vi "lab10.vi"() -> ()   [LabVIEW 2018]
uses:
  <vilib>/measure/NI_MAPro.lvlib
  <vilib>/measure/madcrms.llb/Basic Averaged DC-RMS for 1 Chan.vi
panel:
  out "Waveform Chart":waveform(dbl)(graph)
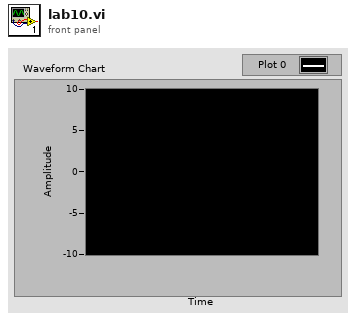
[diagram p1: front panel]
types:
  T1 = enum16{"open", "open or create", "create or replace", "create", "open (read-only)"}
  T2 = cluster{"status":timestamp, "source":string, "Y":dbl[]}
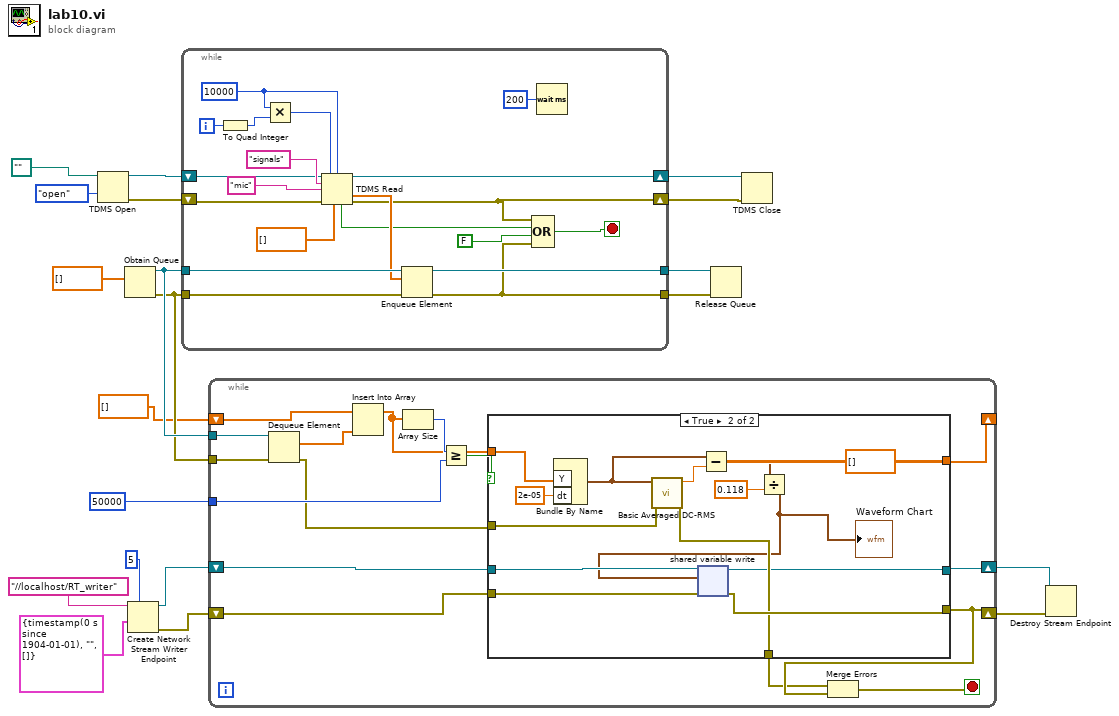
[diagram p0: block diagram]
diagram:
  n1 = TDMS Open(10:T1."open" ("operation (0:open)"), 11:path "" ("file path")) -> (0:w19:errorcluster, 3:w20:refnum<k34>)  [unwired: 5 in]
  n2 = Obtain Queue(element data type=dbl[] [] ("Y")) -> (queue out=w15:refnum<queue>, error out=w14:errorcluster)  [unwired: 4 in, 1 out]
  n3 = Create Network Stream Writer Endpoint(7:5 ("writer buffer size"), 9:T2 {"status"=timestamp(0 s since 1904-01-01), "source"="", "Y"=[]} ("error in (no error)"), 11:"//localhost/RT_writer" ("writer name")) -> (0:w11:errorcluster, 3:w10:refnum<k21>)  [unwired: 4 in]
  n4 = while {
    shift-right: [w21] -> w1
    shift-left: w20 -> [w35]
    shift-right: [w22] -> w2
    shift-left: w19 -> [w33]
    tunnel: w15 -> [w30]
    tunnel: w14 -> [w28]
    tunnel: [w27] -> w17
    tunnel: [w24] -> w16
    i -> [w39]
    stop <- w26 stop-if-true
    w37 = 10000
    n5 = To Quad Integer(1:w39) -> (0:w40:i64)
    n6 = Multiply(x=w37, y=w40) -> (x*y=w38:i64)
    n7 = TDMS Read(0:w35, 1:w38, 2:w37, 5:"signals", 7:"mic", 11:w33, 12:dbl[] [] ("Y")) -> (4:w21:refnum<k34>, 10:w29:dbl[], 14:w25:bool, 15:w22:errorcluster)  [unwired: 1 in, 2 out]
    n8 = Enqueue Element(queue=w30, element=w29, error in (no error)=w28) -> (queue out=w27:refnum<queue>, error out=w24:errorcluster)  [unwired: 1 in, 1 out]
    n9 = Compound Arithmetic op=OR(w22, w25, FALSE ("value"), w24) -> (w26:bool)
    n10 = Wait (ms)(milliseconds to wait=u32 200) -> ()  [unwired: 1 out]
  }
  n11 = while {
    tunnel: w15 -> [w56]
    tunnel: w14 -> [w55]
    shift-right: [w49] -> _
    shift-left: dbl[] [] ("Y") -> [w54]
    tunnel: 50000 -> [w48]
    shift-right: [w44] -> w4
    shift-left: w10 -> [w46]
    shift-right: [w42] -> w3
    shift-left: w11 -> [w43]
    stop <- w45 stop-if-true
    n12 = Dequeue Element(queue=w56, error in (no error)=w55) -> (element=w53:dbl[], error out=w47:errorcluster)  [unwired: 1 in, 2 out]
    n13 = Insert Into Array(array=w54, new element=w53) -> (w50:dbl[])  [unwired: 1 in]
    n14 = Array Size(array=w50) -> (size(s)=w52:i32)
    n15 = Greater Or Equal?(x=w52, y=w48) -> (x >= y?=w51:bool)
    n16 = case shown="True" w51 {
      tunnel: w50 -> [w60 w74]
      tunnel: [w60 dbl[] [] ("Y")] -> w49
      tunnel: w47 -> [w57 w68]
      tunnel: [w58 w66] -> w42
      tunnel: w46 -> [w59 w65]
      tunnel: w43 -> [w58 w64]
      tunnel: [w57 w63] -> w41
      tunnel: [w59 w62] -> w44
      frame False {
      }
      frame True {
        n17 = Bundle By Name("Y"=w74, "dt"=2e-05) -> (w71:waveform(dbl))  [unwired: 1 in]
        n18 = call-poly <vilib>:"Basic Averaged DC-RMS.vi"("error in (no error)"=w68, "signal in"=w71) -> ("error out"=w63:errorcluster, "DC value"=w67:dbl)  [unwired: 6 in, 2 out]
        n19 = Subtract(x=w71, y=w67) -> (x-y=w70:waveform(dbl))
        n20 = Divide(x=w70, y=0.118) -> (x/y=w61:waveform(dbl))
        "Waveform Chart" <- w61
        n21 = shared-variable-write(w65, w64, w61) -> (w62:refnum<k21>, w66:errorcluster)  [unwired: 1 in, 1 out]
      }
    }
    n22 = Merge Errors(w41, w42) -> (w45:errorcluster)
  }
  n23 = Release Queue(queue=w17, error in (no error)=w16) -> ()  [unwired: 1 in, 3 out]
  n24 = TDMS Close(8:w2, 11:w1) -> ()  [unwired: 2 out]
  n25 = Destroy Stream Endpoint(8:w3, 11:w4) -> ()  [unwired: 1 out]
